vi "Read and Write Binary File Examples.vi"() -> ()   [LabVIEW 2015]
panel:
  out "2D Array Data Out":i32[][](array[numeric])
  in  "2D Array Data":i32[][](array[numeric])
  in  "Data":i32
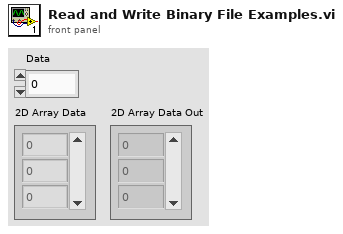
[diagram p1: front panel]
types:
  T1 = enum16{"open", "replace", "create", "open or create", "replace or create", "replace or create with confirmation"}
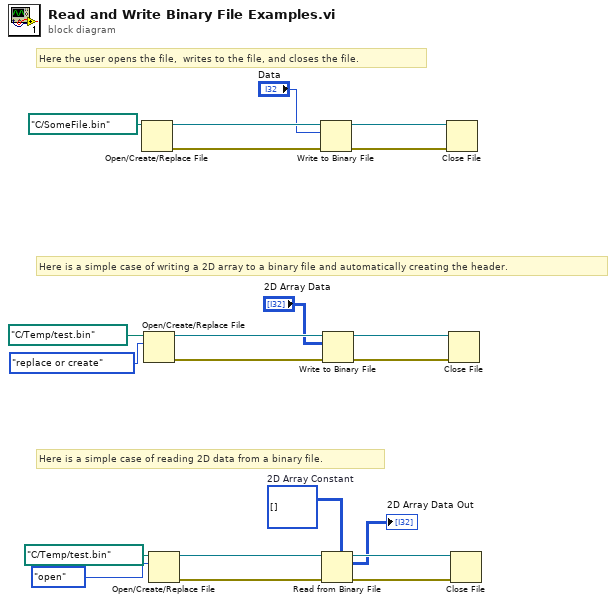
[diagram p0: block diagram]
diagram:
  w1 = i32[][] []  # 2D Array Constant
  # "Here is a simple case of reading 2D data from a binary file."
  # "Here is a simple case of writing a 2D array to a binary file and automatically creating the header."
  # "Here the user opens the file,  writes to the file, and closes the file."
  n1 = Open/Create/Replace File(file path (use dialog)=path "C:/SomeFile.bin") -> (refnum out=w21:refnum<file>, error out=w19:errorcluster)  [unwired: 5 in, 1 out]
  n2 = Open/Create/Replace File(file path (use dialog)=path "C:/Temp/test.bin", operation (0:open)=T1."replace or create") -> (refnum out=w11:refnum<file>, error out=w13:errorcluster)  [unwired: 4 in, 1 out]
  n3 = Open/Create/Replace File(file path (use dialog)=path "C:/Temp/test.bin", operation (0:open)=T1."open") -> (refnum out=w8:refnum<file>, error out=w6:errorcluster)  [unwired: 4 in, 1 out]
  n4 = Write to Binary File(file (use dialog)=w21, data="Data", error in=w19) -> (refnum out=w20:refnum<file>, error out=w18:errorcluster)  [unwired: 3 in, 1 out]
  n5 = Read from Binary File(5:w1, 8:w6, 11:w8) -> (0:w5:errorcluster, 2:→"2D Array Data Out":i32[][], 3:w7:refnum<file>)  [unwired: 3 in, 1 out]
  n6 = Write to Binary File(file (use dialog)=w11, data="2D Array Data", error in=w13) -> (refnum out=w12:refnum<file>, error out=w14:errorcluster)  [unwired: 3 in, 1 out]
  n7 = Close File(refnum=w20, error in=w18) -> ()  [unwired: 2 out]
  n8 = Close File(refnum=w12, error in=w14) -> ()  [unwired: 2 out]
  n9 = Close File(refnum=w7, error in=w5) -> ()  [unwired: 2 out]
